vi "GenerateLines.vi"(10 "Values":dbl[](array[numeric]), 11 "Angles":dbl[](array[numeric])) -> (1 "Intercept":dbl[](array[numeric]), 2 "Slope":dbl[](array[numeric]), 3 "Angles/Indicies":dbl[](array[numeric]))   [LabVIEW 2012]
doc: "This VI takes in a set of angle value pairs as arrays and interpolates lines between them. It outputs arrays of slopes matched with intercepts matched with the indicies of a collection of angles which are used as follows:\n\nTo find a desired angle, iterate through the Angle/Indicies array until the current angle is greater than your desired angle. Then decrement your iterator by one to find the index of your desired slope and intercept.\n\n It works for any angle value pair with an angle input of 0 to 360 degrees. But if you're a stylistic purist don't give it a 0 or 360 degree input: it will still work, but it will have a weird double entry if you look at the output values."
panel:
  out "Numeric":dbl
  # "Inputs"
  # "Outputs"
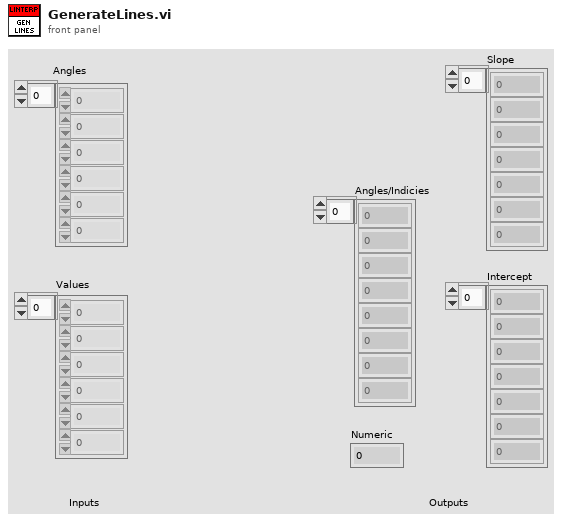
[diagram p1: front panel]
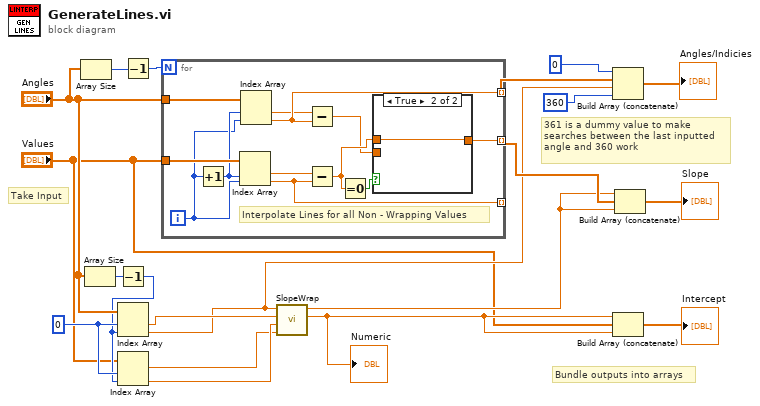
[diagram p0: block diagram]
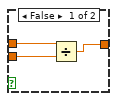
[diagram p2: hidden frame]
diagram:
  w11 = 0
  # "Bundle outputs into arrays"
  # "361 is a dummy value to make\nsearches between the last inputted \nangle and 360 work"
  # "Take Input"
  n1 = Array Size(array="Angles") -> (size(s)=w1:i32)
  n2 = Array Size(array="Angles") -> (size(s)=w6:i32)
  n3 = Decrement(x=w6) -> (x-1=w5:i32)
  n4 = Index Array(array="Angles", index #1=w11, index #2=w5) -> (element #1=w13:dbl, element #2=w7:dbl)
  n5 = Index Array(array="Values", index #1=w11, index #2=w5) -> (element #1=w9:dbl, element #2=w10:dbl)
  n6 = Decrement(x=w1) -> (x-1=w2:i32)
  n7 = for {
    N: w2 -> [_]
    tunnel: "Values" -> [w31]
    tunnel: "Angles" -> [w32]
    tunnel: [w24] -> w15 mode=indexing
    tunnel: [w25] -> _ mode=indexing
    tunnel: [w29] -> w19 mode=indexing
    i -> [w26]
    # "Interpolate Lines for all Non - Wrapping Values"
    n8 = Increment(x=w26) -> (x+1=w30:i32)
    n9 = Index Array(array=w31, index #1=w30, index #2=w26) -> (element #1=w27:dbl, element #2=w25:dbl)
    n10 = Index Array(array=w32, index #1=w30, index #2=w26) -> (element #1=w28:dbl, element #2=w29:dbl)
    n11 = Subtract(x=w28, y=w29) -> (x-y=w21:dbl)
    n12 = Subtract(x=w27, y=w25) -> (x-y=w22:dbl)
    n13 = Equal To 0?(x=w22) -> (x = 0?=w23:bool)
    n14 = case shown="True" w23 {
      tunnel: w21 -> [w34 _]
      tunnel: w22 -> [w35 w36]
      tunnel: [w33 w36] -> w24
      frame False {
        n15 = Divide(x=w35, y=w34) -> (x/y=w33:dbl)
      }
      frame True {
      }
    }
  }
  n16 = call "SlopeWrap.vi"("Low Value"=w9, "High Value"=w10, "Low Angle"=w13, "High Angle"=w7) -> ("0/360 Intercept"=w4:dbl, "Slope"=w14:dbl)  [unwired: 6 in]
  "Numeric" <- w4
  n17 = Build Array (concatenate)(0, w19, w7, 360) -> (→"Angles/Indicies":dbl[])
  n18 = Build Array (concatenate)(w4, "Values", w4) -> (→"Intercept":dbl[])
  n19 = Build Array (concatenate)(w14, w15, w14) -> (→"Slope":dbl[])
